vi "Test Asic Rate Scan.vi"(8 "Error IN":errorcluster, 11 "Config Test IN":T2 {"CONFIG GEN"."Vasic Theorical" min=1.0 max=1000000.0 step=1.0 format="%#_6pV"; "CONFIG GEN"."Frequency" min=0.001 max=333000000.0 step=1000.0 format="%#_6pHz"; "CONFIG GEN"."Leading Edge Time" min=1e-09 max=1.0 step=1e-10 format="%#_6ps"; "CONFIG GEN"."Trailing Edge Time" min=1e-09 max=1.0 step=1e-10 format="%#_6ps"; "CONFIG GEN"."Delay" min=0.0 max=1.0 step=1e-12 format="%#_6ps"; "CONFIG GEN"."Trigger Level Sync" items=["ECL", "TTL"]; "CONFIG GEN"."Trigger Sync Out" items=["AB"=3, "B"=2, "A"=1, "None"=0]; "CONFIG GEN"."Load" min=1.0 max=1000000.0 step=1.0 format="%#_6p"; "CONFIG GEN"."DC Offset" min=-10.0 max=10.0 step=0.1 format="%#_6pV"; "CONFIG GEN"."Amplitude" min=0.05 max=5.0 step=0.001 format="%#_6pV"; "CONFIG GEN"."Width Time" min=1.5e-09 max=1.0 step=1e-10 format="%#_6ps"; "CONFIG GEN"."Channel" items=["Channel1"=1, "Channel2"=2]; "Config VGA"."Theoretical Voltage" format="%1.4f"; "Config VGA"."VGA Gain" format="%02x"; "Config VGA"."Frecuency Pulse" format="%0_2p"; "Config VGA"."Pulse Width" format="%04x"; "Config VGA"."Real Voltage" format="%1.5f"; "Config Test"."VALUE IBIAS" max=63 step=1; "Config Test"."Vasic real f.a." min=2.8 max=3.8 step=0.01 format="%.2g"; "Config Test"."Limits Rate Scan adders"."Low" format="%1.3f"; "Config Test"."Limits Rate Scan adders"."High" format="%1.3f"; "Config Test"."Limits ADC"."High" format="%1.4f"; "Config Test"."Limits ADC"."Low" format="%1.3f"; "Config Test"."Lim offset Dig"."Max Dig" format="%.3g"; "Config Test"."Lim Offset Analog"."Min Analog" format="%.3g"; "Config Test"."Lim Offset Analog"."Max Analog" format="%.3g"; "Config Test"."Limits Rate Scan"."Low" format="%1.4f"; "Config Test"."Limits Rate Scan"."High" format="%1.3f"; "Config Test"."Limits Max PN Min NP"."Min P Upper" format="%.3g"; "Config Test"."Limits Max PN Min NP"."Min P Lower" format="%.3g"; "Config Test"."Limits Max PN Min NP"."Max N Lower" format="%.3g"; "Config Test"."Limits Max PN Min NP"."Max N Upper" format="%.3g"; "Config Test"."Limits Max PN Min NP"."Min N Lower" format="%.3g"; "Config Test"."Limits Max PN Min NP"."Min N Upper" format="%.3g"; "Config Test"."Limits Max PN Min NP"."Max P Upper" format="%.3g"; "Config Test"."Limits Max PN Min NP"."Max P Lower" format="%.3g"; "Config Test"."Vasic" min=2.8 max=3.8 step=0.01 format="%.2g"; "Config HW"."Config Rigol DP832"."Channel" items=["+30V Channel 1", "+30V Channel 2", "+5V Channel 3"]; "Config HW"."Config Rigol DP832"."V Limit" format="%.1g"; "Config HW"."Config Rigol DP832"."I Limit" format="%.1g"; "Config HW"."Config Rigol DP832"."V Out" format="%.1g"; "Result"."Test Registros"."Read W/R" format="%04x"; "Result"."Test Registros"."Pattern W/R" format="%04x"; "Result"."Test Registros"."Read Default" format="%04x"; "Result"."Test Registros"."Pattern Default" format="%04x"}) -> (0 "Error OUT":errorcluster={"status"=TRUE, "code"=-1073807343, "source"="VISA Write in Tektronix DPO MSO 2000 4000 Series.lvlib:Auto Scale Math Waveform.vi->TEK_Configura formula Math.vi->Configure osciloscopio FULL con generador.vi->Test Asic Rate Scan.vi->Test Asic V1.0 - copia2019.vi"}, 2 "Rate scan all ok":bool, 3 "Config Test OUT":T2 {"CONFIG GEN"."Vasic Theorical" min=1.0 max=1000000.0 step=1.0 format="%#_6pV"; "CONFIG GEN"."Frequency" min=0.001 max=333000000.0 step=1000.0 format="%#_6pHz"; "CONFIG GEN"."Leading Edge Time" min=1e-09 max=1.0 step=1e-10 format="%#_6ps"; "CONFIG GEN"."Trailing Edge Time" min=1e-09 max=1.0 step=1e-10 format="%#_6ps"; "CONFIG GEN"."Delay" min=0.0 max=1.0 step=1e-12 format="%#_6ps"; "CONFIG GEN"."Trigger Level Sync" items=["ECL", "TTL"]; "CONFIG GEN"."Trigger Sync Out" items=["AB"=3, "B"=2, "A"=1, "None"=0]; "CONFIG GEN"."Load" min=1.0 max=1000000.0 step=1.0 format="%#_6p"; "CONFIG GEN"."DC Offset" min=-10.0 max=10.0 step=0.1 format="%#_6pV"; "CONFIG GEN"."Amplitude" min=0.05 max=5.0 step=0.001 format="%#_6pV"; "CONFIG GEN"."Width Time" min=1.5e-09 max=1.0 step=1e-10 format="%#_6ps"; "CONFIG GEN"."Channel" items=["Channel1"=1, "Channel2"=2]; "Config VGA"."Theoretical Voltage" format="%1.4f"; "Config VGA"."VGA Gain" format="%02x"; "Config VGA"."Frecuency Pulse" format="%0_2p"; "Config VGA"."Pulse Width" format="%04x"; "Config VGA"."Real Voltage" format="%1.5f"; "Config Test"."VALUE IBIAS" max=63 step=1; "Config Test"."Vasic real f.a." min=2.8 max=3.8 step=0.01 format="%.2g"; "Config Test"."Limits Rate Scan adders"."Low" format="%1.3f"; "Config Test"."Limits Rate Scan adders"."High" format="%1.3f"; "Config Test"."Limits ADC"."High" format="%1.4f"; "Config Test"."Limits ADC"."Low" format="%1.3f"; "Config Test"."Lim offset Dig"."Max Dig" format="%.3g"; "Config Test"."Lim Offset Analog"."Min Analog" format="%.3g"; "Config Test"."Lim Offset Analog"."Max Analog" format="%.3g"; "Config Test"."Limits Rate Scan"."Low" format="%1.4f"; "Config Test"."Limits Rate Scan"."High" format="%1.3f"; "Config Test"."Limits Max PN Min NP"."Min P Upper" format="%.3g"; "Config Test"."Limits Max PN Min NP"."Min P Lower" format="%.3g"; "Config Test"."Limits Max PN Min NP"."Max N Lower" format="%.3g"; "Config Test"."Limits Max PN Min NP"."Max N Upper" format="%.3g"; "Config Test"."Limits Max PN Min NP"."Min N Lower" format="%.3g"; "Config Test"."Limits Max PN Min NP"."Min N Upper" format="%.3g"; "Config Test"."Limits Max PN Min NP"."Max P Upper" format="%.3g"; "Config Test"."Limits Max PN Min NP"."Max P Lower" format="%.3g"; "Config Test"."Vasic" min=2.8 max=3.8 step=0.01 format="%.2g"; "Config HW"."Config Rigol DP832"."Channel" items=["+30V Channel 1", "+30V Channel 2", "+5V Channel 3"]; "Config HW"."Config Rigol DP832"."V Limit" format="%.1g"; "Config HW"."Config Rigol DP832"."I Limit" format="%.1g"; "Config HW"."Config Rigol DP832"."V Out" format="%.1g"; "Result"."Test Registros"."Read W/R" format="%04x"; "Result"."Test Registros"."Pattern W/R" format="%04x"; "Result"."Test Registros"."Read Default" format="%04x"; "Result"."Test Registros"."Pattern Default" format="%04x"})   [LabVIEW 2019]
uses:
  Test.ctl
  TEST.TEST CONFIG HW.ctl
  Rigol DP832/DP832_Control Channels.ctl
  TEST.TEST CONFIG TEST MATRIZ.ctl
  TEST.TEST CONFIG TEST.ctl
  TEST.TEST RESULT.ctl
  test_result fvasic.ctl
  TEST.TEST EXECUTION TEST.ctl
  TEST.TEST CONFIG VGA.ctl
  TEST.TEST TEST INFO.ctl
  TEST.TEST INFO PC.ctl
  GenPulse_configurar.ctl
  Global.Salir Ya.vi
panel:
  in  "VISA Tek MDO3104":refnum<visa-resource-name>="USB0::0x0699::0x0408::C016316::INSTR"
  in  "Debug":enum32{"Page 1", "Page 2"}(tab)
  in  "Operacion":enum32{"Page 1", "Page 2"}(tab)
  out "%":u8=9 format="%02d%%"
  out "B":u8(slide)=9 scale=0.0..100.0
  out "Indicador":string="VTheo 0,0500V (Vreal 0,0000V)\nChannel 7 Adder C\nTotal Errors: 0"
  out "Amplitude":dbl
  out "HLTHx":dbl
  out "LLTHx":dbl
  out "WRITE OK":bool
  out "DAC TH0,TH1,TH2 2":u16[][][](array[numeric])
  out "DAC TH3,TH4,TH5 2":u16[][][](array[numeric])
  out "Volt HLTH (salida A)":dbl[][][](array[numeric])
  out "Volt LLTH (salida B)":dbl[][][](array[numeric])
  out "DAC TH0,TH1,TH2":u16
  out "DAC TH3,TH4,TH5":u16
  out "Reference":T1={"Sumador"=2, "Canal"=6, "Tension"=0, "Tension Real"=0.0}
  out "Comparation HLTH":bool[][][](array[boolean])
  out "Comparation LLTH":bool[][][](array[boolean])
  out "Volt HLTH (salida A) corregida":dbl[][][](array[numeric])=[[[nan, nan, nan], [nan, nan, nan], [nan, nan, nan], [nan, nan, nan], [nan, nan, nan], [nan, nan, nan], [nan, nan, nan]]]
  out "HLTH (salida A) cruce por 0":dbl[][](array[numeric])=[[nan, nan, nan], [nan, nan, nan], [nan, nan, nan], [nan, nan, nan], [nan, nan, nan], [nan, nan, nan], [nan, nan, nan]]
  out "Volt LLTH (salida b) corregida":dbl[][][](array[numeric])=[[[nan, nan, nan], [nan, nan, nan], [nan, nan, nan], [nan, nan, nan], [nan, nan, nan], [nan, nan, nan], [nan, nan, nan]]]
  out "LLTH (salida b) cruce por 0":dbl[][](array[numeric])=[[nan, nan, nan], [nan, nan, nan], [nan, nan, nan], [nan, nan, nan], [nan, nan, nan], [nan, nan, nan], [nan, nan, nan]]
  out "HIGH":dbl[](array[numeric])=[0.0593, 0.1073, 0.2039, 0.2977, 0.3918, 0.4828, 0.5702, 0.6594, 0.7367, 0.8087, 0.867]
  out "loW":dbl[](array[numeric])=[0.0264, 0.0665, 0.1423, 0.2207, 0.2962, 0.3691, 0.4392, 0.5107, 0.5726, 0.6304, 0.6771]
  out "Vin asic Theo":dbl[](array[numeric])=[0.05, 0.1, 0.2, 0.3, 0.4, 0.51, 0.6, 0.7, 0.8, 0.9, 1.0]
  out "Vin real gen":dbl[](array[numeric])=[0.054, 0.106, 0.216, 0.322, 0.43, 0.538, 0.648, 0.752, 0.86, 0.966, 1.076]
  # "Vin Asic"
  # "CANAL"
  # "Canal"
  # "VIN ASIC"
  # "Sumador"
  # "Vin Asic"
  # "CANAL"
  # "Canal"
  # "VIN ASIC"
  # "Sumador"
  # "Test ASIC. Rate Scan"
  # "Modo 2\nModo 3\nModo 4\nModo 2\nModo 3\nModo 4"
  # "Modo 2\nModo 3\nModo 4\nModo 2\nModo 3\nModo 4"
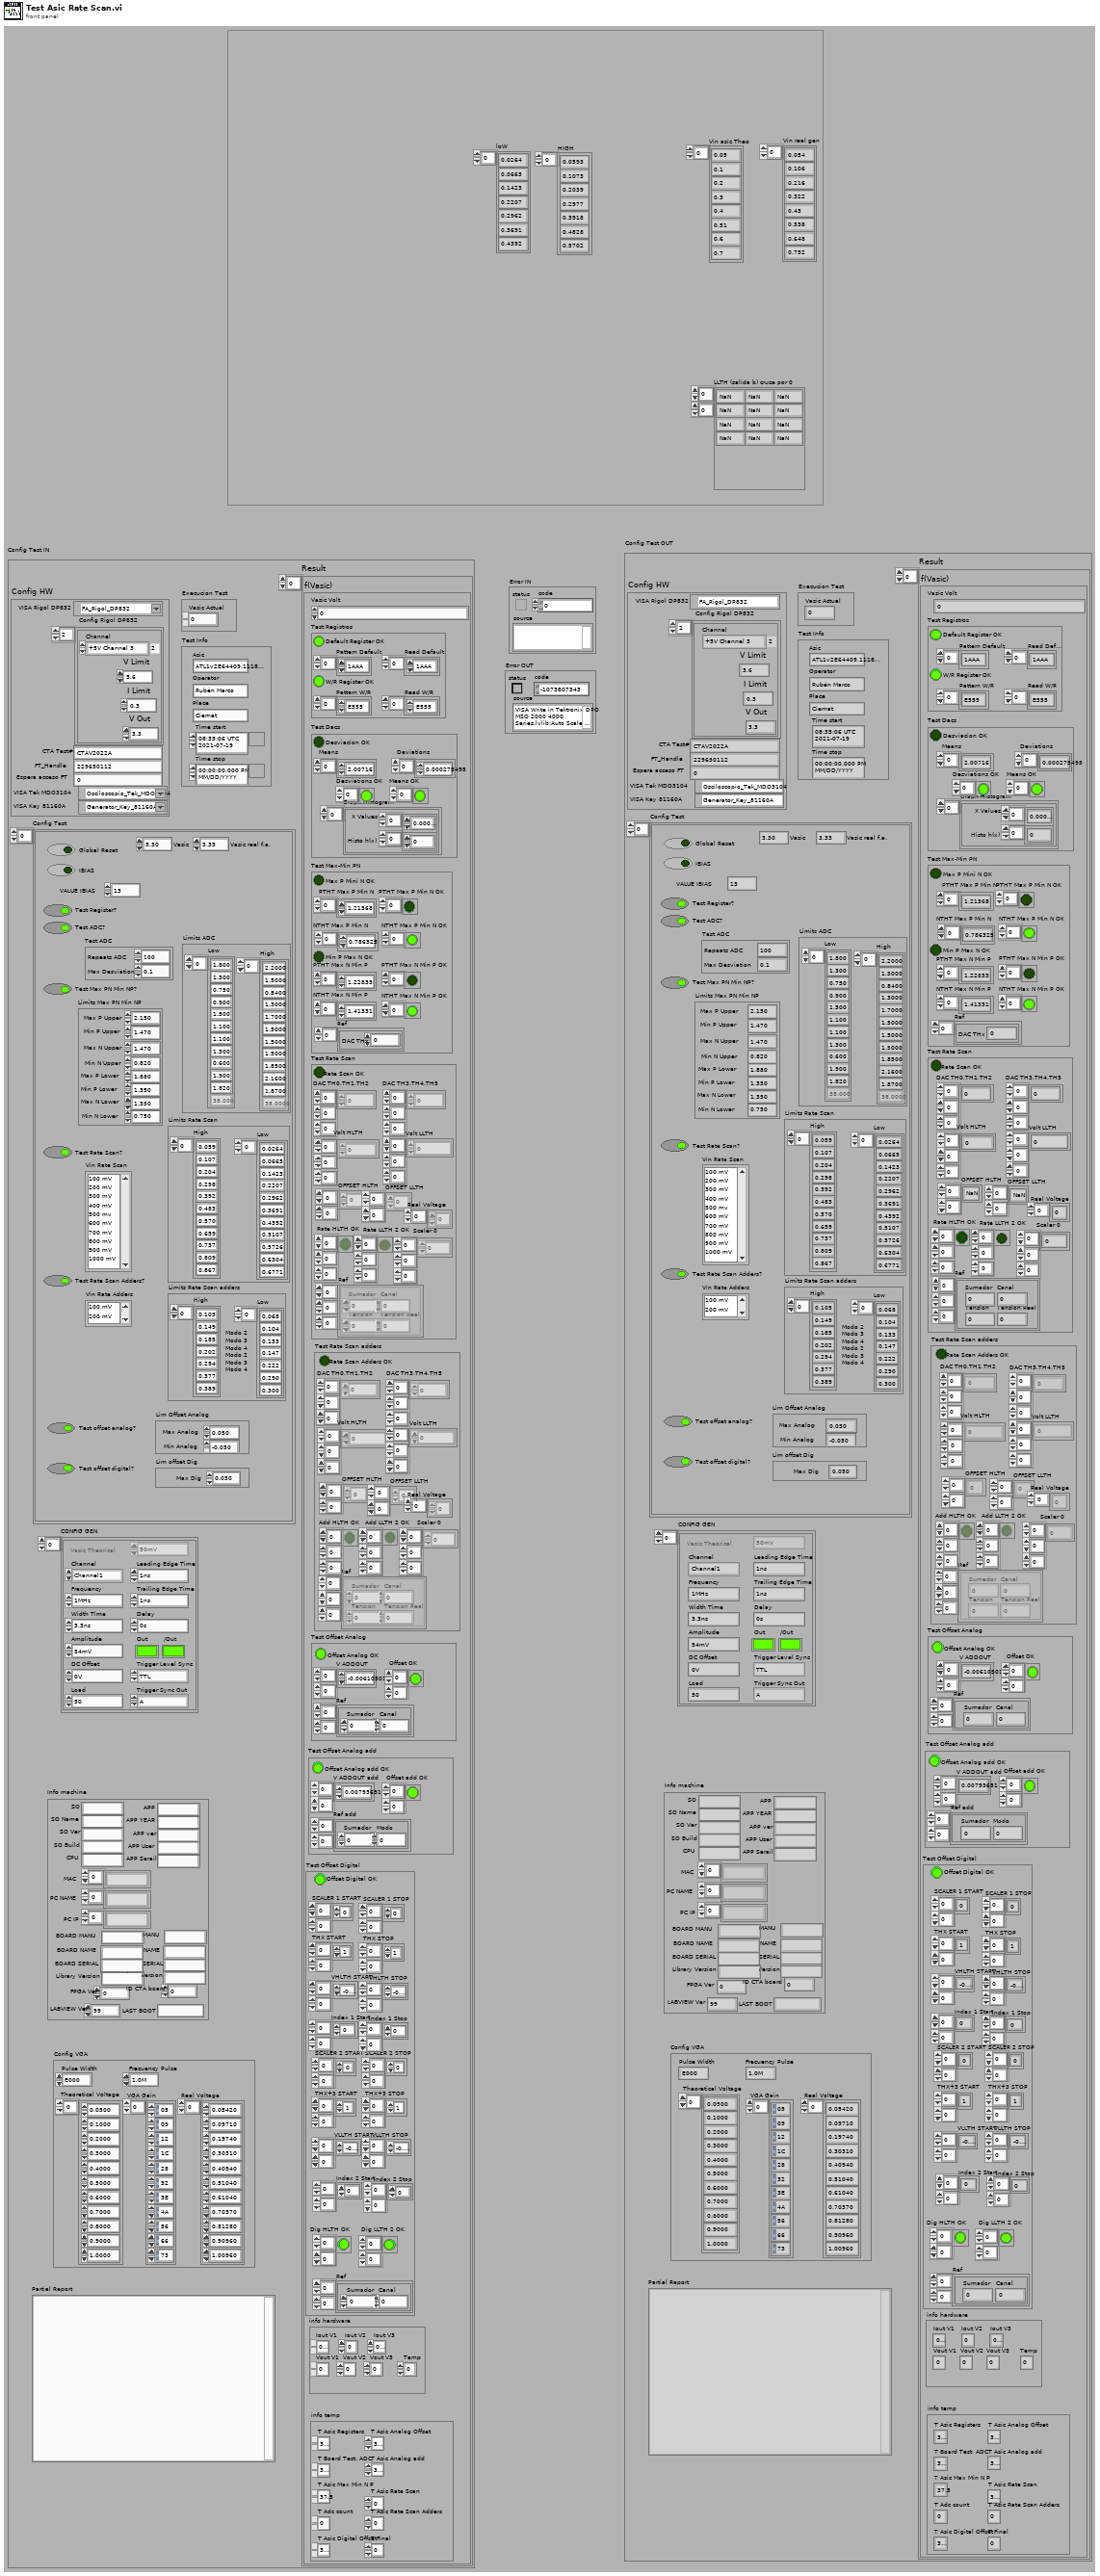
[diagram p1: front panel]
types:
  T1 = cluster{"Sumador":u8, "Canal":u8, "Tension":u8, "Tension Real":dbl}
  T2 = typedef "Test.ctl" = cluster{"Config HW":T3, "Config Test":T5, "Result":T7, "Execucion Test":T9, "Config VGA":T10, "Test Info":T11, "Info machine":T12, "Partial Report":string, "CONFIG GEN":T13[]}
  T3 = typedef "TEST.TEST CONFIG HW.ctl" = cluster{"VISA Rigol DP832":refnum<visa-resource-name>, "Config Rigol DP832":cluster{"Channel":T4, "V Limit":dbl, "I Limit":dbl, "V Out":dbl}[], "CTA Test#":string, "FT_Handle":u32, "Espera acceso FT":u32, "VISA Tek MDO3104":refnum<visa-resource-name>, "VISA Key 81160A":refnum<visa-resource-name>}
  T4 = typedef "DP832_Control Channels.ctl" = i32
  T5 = typedef "TEST.TEST CONFIG TEST MATRIZ.ctl" = T6[]
  T6 = typedef "TEST.TEST CONFIG TEST.ctl" = cluster{"Vasic":dbl, "Global Reset":bool, "Test Register?":bool, "Test ADC?":bool, "Test ADC":cluster{"Repeats ADC":i32, "Max Desviation":dbl}, "Limits ADC":cluster{"Low":dbl[], "High":dbl[]}, "Test Max PN Min NP?":bool, "Limits Max PN Min NP":cluster{"Max P Upper":dbl, "Min P Upper":dbl, "Max N Upper":dbl, "Min N Upper":dbl, "Max P Lower":dbl, "Min P Lower ":dbl, "Max N Lower":dbl, "Min N Lower":dbl}, "Test Rate Scan?":bool, "Vin Rate Scan":i32[], "Limits Rate Scan":cluster{"High":dbl[], "Low":dbl[]}, "Test Rate Scan Adders?":bool, "Vin Rate Adders":i32[], "Limits Rate Scan adders":cluster{"High":dbl[], "Low":dbl[]}, "Test offset analog?":bool, "Lim Offset Analog":cluster{"Max Analog":dbl, "Min Analog":dbl}, "Test offset digital?":bool, "Lim offset Dig":cluster{"Max Dig":dbl}, "Vasic real f.a.":dbl, "IBIAS":bool, "VALUE IBIAS":u8}
  T7 = typedef "TEST.TEST RESULT.ctl" = T8[]
  T8 = typedef "test_result fvasic.ctl" = cluster{"Vasic Volt":i32, "Test Registros":cluster{"Default Register OK":bool, "Pattern Default":u16[], "Read Default":u16[], "W/R Register OK":bool, "Pattern W/R":u16[], "Read W/R":u16[]}, "Test Dacs":cluster{"Desviacion OK":bool, "Means":dbl[], "Deviations":dbl[], "Desviations OK":bool[], "Means OK":bool[], "Graph Histogram":cluster{"X Values":dbl[], "Histo h(x)":i32[]}[]}, "Test Max-Min PN":cluster{"Max P Mini N OK":bool, "PTHT Max P Min N":dbl[], "PTHT Max P Min N OK":bool[], "NTHT Max P Min N":dbl[], "NTHT Max P Min N OK":bool[], "Min P Max N OK":bool, "PTHT Max N Min P":dbl[], "PTHT Max N Min P OK":bool[], "NTHT Max N Min P":dbl[], "NTHT Max N Min P OK":bool[], "Ref":cluster{"DAC THx":u8}[]}, "Test Rate Scan":cluster{"Rate Scan OK":bool, "DAC TH0,TH1,TH2":u16[][][], "Volt HLTH":dbl[][][], "Rate HLTH OK":bool[][][], "DAC TH3,TH4,TH5":u16[][][], "Volt LLTH":dbl[][][], "Rate LLTH 2 OK":bool[][][], "Scaler 0":u16[][][], "Ref":cluster{"Sumador":u8, "Canal":u8, "Tension":u8, "Tension Real":dbl}[][][], "OFFSET HLTH":dbl[][], "OFFSET LLTH":dbl[][], "Real Voltage":dbl[]}, "Test Rate Scan adders":cluster{"Rate Scan Adders OK":bool, "DAC TH0,TH1,TH2":u16[][][], "Volt HLTH":dbl[][][], "Add HLTH OK":bool[][][], "DAC TH3,TH4,TH5":u16[][][], "Volt LLTH":dbl[][][], "Add LLTH 2 OK":bool[][][], "Scaler 0":u16[][][], "Ref":cluster{"Sumador":u8, "Canal":u8, "Tension":u8, "Tension Real":dbl}[][][], "OFFSET HLTH":dbl[][], "OFFSET LLTH":dbl[][], "Real Voltage":dbl[]}, "Test Offset Analog":cluster{"Offset Analog OK":bool, "V ADDOUT":dbl[][], "Offset OK":bool[][], "Ref":cluster{"Sumador":u8, "Canal":u8}[][]}, "Test Offset Digital":cluster{"Offset Digital OK":bool, "SCALER 1 START":u16[][], "SCALER 1 STOP":u16[][], "THX START":u16[][], "THX STOP":u16[][], "VHLTH START":dbl[][], "VHLTH STOP":dbl[][], "Index 1 Start":i32[][], "index 1 Stop":i32[][], "SCALER 2 START":u16[][], "SCALER 2 STOP":u16[][], "THX+3 START":u16[][], "THX+3 STOP":u16[][], "VLLTH START":dbl[][], "VLLTH STOP":dbl[][], "Index 2 Start":i32[][], "index 2 Stop":i32[][], "Dig HLTH OK":bool[][], "Dig LLTH 2 OK":bool[][], "Ref":cluster{"Sumador":u8, "Canal":u8}[][]}, "info hardware":cluster{"Iout V1":dbl, "Iout V2":dbl, "Iout V3":dbl, "Vout V1":dbl, "Vout V2":dbl, "Vout V3":dbl, "Temp":dbl}, "Test Offset Analog add":cluster{"Offset Analog add OK":bool, "V ADDOUT add":dbl[][], "Offset add OK":bool[][], "Ref add":cluster{"Sumador":u8, "Modo":u8}[][]}, "info temp":cluster{"T Asic Registers":dbl, "T Board Test. ADC":dbl, "T Asic Max Min N P":dbl, "T Adc count":dbl, "T Asic Digital Offset":dbl, "T Asic Analog Offset":dbl, "T Asic Analog add":dbl, "T Asic Rate Scan":dbl, "T Asic Rate Scan Adders":dbl, "T Final":dbl}}
  T9 = typedef "TEST.TEST EXECUTION TEST.ctl" = cluster{"Vasic Actual":i32}
  T10 = typedef "TEST.TEST CONFIG VGA.ctl" = cluster{"Theoretical Voltage":dbl[], "Real Voltage":dbl[], "Pulse Width":u16, "Frecuency Pulse":dbl, "VGA Gain":u8[]}
  T11 = typedef "TEST.TEST TEST INFO.ctl" = cluster{"Asic":string, "Operator":string, "Place":string, "Time start":timestamp, "Time stop":timestamp}
  T12 = typedef "TEST.TEST INFO PC.ctl" = cluster{"SO":string, "SO Name":string, "SO Ver":string, "SO Build":string, "CPU":string, "APP":string, "APP YEAR":string, "APP ver":string, "APP User":string, "APP Serail":string, "MAC":string[], "PC NAME":string[], "PC IP":string[], "BIOS MANU":string, "BIOS NAME":string, "BIOS SERIAL":string, "BOARD MANU":string, "BOARD NAME":string, "BOARD SERIAL":string, "Driver Version":string, "Library Version":string, "FPGA Ver":u8, "ID CTA board":u64, "LAST BOOT":string, "LABVIEW Ver":u32}
  T13 = typedef "GenPulse_configurar.ctl" = cluster{"Channel":u16, "Frequency":dbl, "Width Time":dbl, "Amplitude":dbl, "DC Offset":dbl, "Load":dbl, "Leading Edge Time":dbl, "Trailing Edge Time":dbl, "Delay":dbl, "Out":bool, "/Out":bool, "Trigger Level Sync":u16, "Trigger Sync Out":u16, "Vasic Theorical":dbl}
  T14 = enum16{"Always On", "Always Off", "Off While Running"}
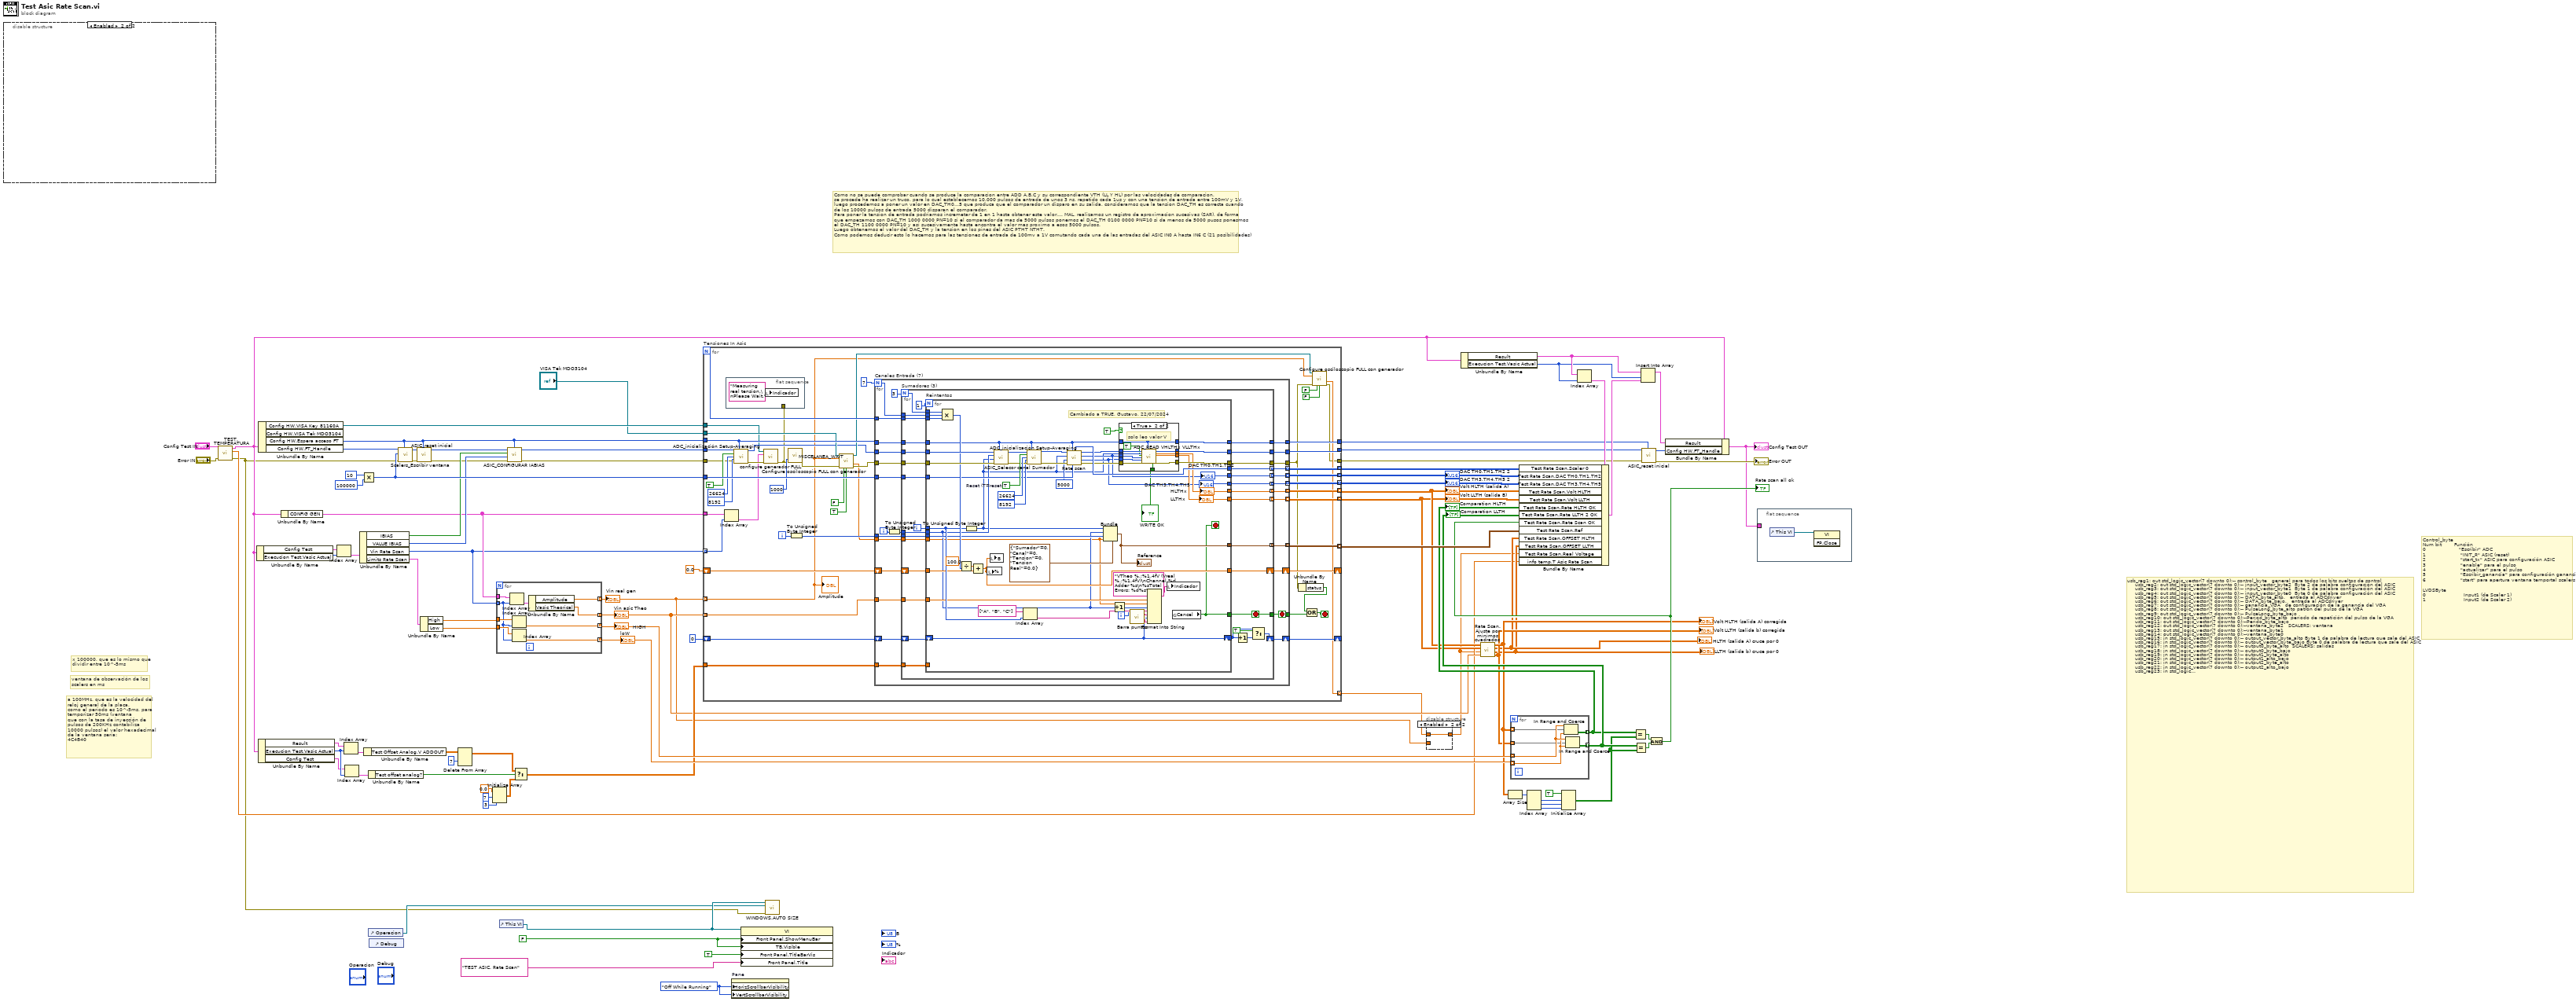
[diagram p0: block diagram]
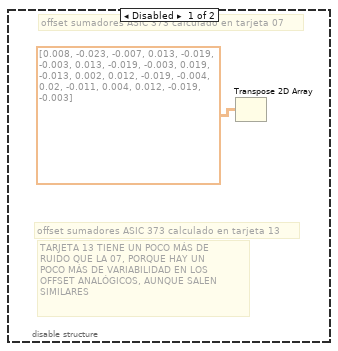
[diagram p3: hidden frame]
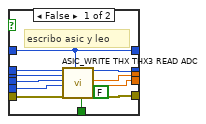
[diagram p4: hidden frame]
diagram:
  w22 = T14."Off While Running" ("Horizontal Scrollbar Visibility")
  w53 = FALSE ("Front Panel Window:Show Menu Bar")
  # "Como no se puede comprobar cuando se produce la comparacion entre ADD A,B,C y su correspondiente VTH (LL Y HL) por las velocidades de comparacion,\nse procede ha realizar un truco, para lo cual establecemos 10.000 pulsos de entrada de unos 3 ns, repetido cada 1us y con una tension de entrada entre 100mV y 1V,\nluego procedemos a poner un valor en DAC_TH0...5 que produca que el comparador un disparo en su salida, consideramos que la tension DAC_TH es correcta cuando\nde los 10000 pulsos de entrada 5000 disparan el comparador.\nPara poner la tension de entrada podriamos incremetar de 1 en 1 hasta obtener este valor.... MAL. realizamos un registro de aproximacion sucesivas (SAR), de forma\nque empezamos con DAC_TH 1000 0000 PN=10 si el comparador da mas de 5000 pulsos ponemos el DAC_TH 0100 0000 PN=10 si da menos de 5000 pusos ponesmos\nel DAC_TH 1100 0000 PN=10 y asi sucesivamente hasta encontra el valor mas proximo a esos 5000 pulsos. \nLuego obtenemos el valor del DAC_TH y la tension en los pines del ASIC PTHT NTHT.\nComo podemos deducir esto lo hacemos para las tensiones de entrada de 100mv a 1V comutando cada una de las entradas del ASIC IN0 A hasta IN6 C (21 posibilidades)"
  # "Control_byte\nNum bit        Función\n0                     \"Escribir\" ADC\n1                      \"INIT_R\" ASIC (reset)\n2                      \"start_tx\" ASIC para configuración ASIC\n3                      \"enable\" para el pulso\n4                      \"actualizar\" para el pulso\n5                      \"Escribir_ganancia\" para configuración ganancia\n6                      \"start\" para apertura ventana temportal scalers\n\nLVDSByte\n0                        Input1 (de Scaler 1)\n1                        Input2 (de Scaler 2)"
  # "usb_reg1: out std_logic_vector(7 downto 0);-- control_byte\t\t\tgeneral para todos los bits sueltos de control\n\t\t\t  usb_reg2: out std_logic_vector(7 downto 0);-- input_vector_byte2 \tByte 2 de palabra configuración del ASIC\n\t\t\t  usb_reg3: out std_logic_vector(7 downto 0);-- input_vector_byte1 \tByte 1 de palabra configuración del ASIC\n\t\t\t  usb_reg4: out std_logic_vector(7 downto 0);-- input_vector_byte0 \tByte 0 de palabra configuración del ASIC\n\t\t\t  usb_reg5: out std_logic_vector(7 downto 0);-- DATA_byte_alto, \t\tentrada al ADCdriver\n\t\t\t  usb_reg6: out std_logic_vector(7 downto 0);-- DATA_byte_bajo, \t\tentrada al ADCdriver\n\t\t\t  usb_reg7: out std_logic_vector(7 downto 0);-- ganancia_VGA\t\t\tde configuración de la ganancia del VGA\n\t\t\t  usb_reg8: out std_logic_vector(7 downto 0);-- PulseLong_byte_alto\tpatrón del pulso de la VGA\n\t\t\t  usb_reg9: out std_logic_vector(7 downto 0);-- PulseLong_byte_bajo\n\t\t\t  usb_reg10: out std_logic_vector(7 downto 0);--Period_byte_alto\t\tperíodo de repetición del pulso de la VGA\n\t\t\t  usb_reg11: out std_logic_vector(7 downto 0);--Perido_byte_bajo\n\t\t\t  usb_reg12: out std_logic_vector(7 downto 0);--ventana_byte2\t\t\tSCALERS: ventana\n\t\t\t  usb_reg13: out std_logic_vector(7 downto 0);--ventana_byte1\t\n\t\t\t  usb_reg14: out std_logic_vector(7 downto 0);--ventana_byte0\n\t\t\t  usb_reg15: in std_logic_vector(7 downto 0);-- output_vector_byte_alto\tByte 1 de palabra de lectura que sale del ASIC\n\t\t\t  usb_reg16: in std_logic_vector(7 downto 0);-- output_vector_byte_bajo\tByte 0 de palabra de lectura que sale del ASIC\n\t\t\t  usb_reg17: in std_logic_vector(7 downto 0);-- output0_byte_alto\t\tSCALERS: salidas\n\t\t\t  usb_reg18: in std_logic_vector(7 downto 0);-- output0_byte_bajo\n\t\t\t  usb_reg19: in std_logic_vector(7 downto 0);-- output1_byte_alto\n\t\t\t  usb_reg20: in std_logic_vector(7 downto 0);-- output1_alto_bajo \n\t\t\t  usb_reg21: in std_logic_vector(7 downto 0);-- output2_byte_alto \n\t\t\t  usb_reg22: in std_logic_vector(7 downto 0);-- output2_alto_bajo \n\t\t\t  usb_reg23: in std_logic_vector(7 downto 0);-- para el canal_0 del ADCdriver\n\t\t\t  usb_reg24: in std_logic_vector(7 downto 0);\n\t\t\t  usb_reg25: in std_logic_vector(7 downto 0);-- para el canal_1 del ADCdriver\n\t\t\t  usb_reg26: in std_logic_vector(7 downto 0);\n\t\t\t  usb_reg27: in std_logic_vector(7 downto 0);-- para el canal_2 del ADCdriver\n\t\t\t  usb_reg28: in std_logic_vector(7 downto 0);\n\t\t\t  usb_reg29: in std_logic_vector(7 downto 0);-- para el canal_3 del ADCdriver\n\t\t\t  usb_reg30: in std_logic_vector(7 downto 0);\n\t\t\t  usb_reg31: in std_logic_vector(7 downto 0);-- para el canal_4 del ADCdriver\n\t\t\t  usb_reg32: in std_logic_vector(7 downto 0);\n\t\t\t  usb_reg33: in std_logic_vector(7 downto 0);-- para el canal_5 del ADCdriver\n\t\t\t  usb_reg34: in std_logic_vector(7 downto 0);\n\t\t\t  usb_reg35: in std_logic_vector(7 downto 0);-- para el canal_6 del ADCdriver\n\t\t\t  usb_reg36: in std_logic_vector(7 downto 0);\n\t\t\t  usb_reg37: in std_logic_vector(7 downto 0);-- para el canal_7 del ADCdriver\n\t\t\t  usb_reg38: in std_logic_vector(7 downto 0);\n\t\t\t  usb_reg39: in std_logic_vector(7 downto 0);-- para el canal_8 del ADCdriver\n\t\t\t  usb_reg40: in std_logic_vector(7 downto 0);\n\t\t\t  usb_reg41: in std_logic_vector(7 downto 0);-- para el canal_9 del ADCdriver\n\t\t\t  usb_reg42: in std_logic_vector(7 downto 0);\n\t\t\t  usb_reg43: in std_logic_vector(7 downto 0);-- para el canal_10 del ADCdriver\n\t\t\t  usb_reg44: in std_logic_vector(7 downto 0)--;  \n\n     usb_reg55 => LVDSByte"
  # "x 100000, que es lo mismo que dividir entre 10^-5ms"
  # "ventana de observación de los scalers en ms"
  # "a 100MHz, que es la velocidad del reloj general de la placa,\ncomo el período es 10^-5ms, para temporizar 50ms (ventana \nque con la tasa de inyección de pulsos de 200KHz contabiliza \n10000 pulsos) el valor hexadecimal de la ventana sería:\n4C4B40"
  n1 = disable-structure shown="Enabled" {
    frame Disabled {
      # "TARJETA 13 TIENE UN POCO MÁS DE \nRUIDO QUE LA 07, PORQUE HAY UN\nPOCO MÁS DE VARIABILIDAD EN LOS \nOFFSET ANALÓGICOS, AUNQUE SALEN\nSIMILARES"
      # "offset sumadores ASIC 373 calculado en tarjeta 13"
      # "offset sumadores ASIC 373 calculado en tarjeta 07"
      n2 = Transpose 2D Array(2D array=dbl[][] [[0.008, -0.023, -0.007], [0.013, -0.019, -0.003], [0.013, -0.019, -0.003], [0.019, -0.013, 0.002], [0.012, -0.019, -0.004], [0.02, -0.011, 0.004], [0.012, -0.019, -0.003]]) -> ()  [unwired: 1 out]
    }
    frame Enabled {
    }
  }
  n3 = call "TEST.TEMPERATURA.vi"("error IN"="Error IN", "input cluster"="Config Test IN") -> ("error out"=w4:errorcluster, "Temperatura"=w10:dbl, "OUT cluster 2"=w11:T2)  [unwired: 7 in]
  n4 = Unbundle By Name(w11) -> ("Config Test"=w76:T5, "Execucion Test.Vasic Actual"=w75:i32)
  n5 = Unbundle By Name(w11) -> ("Result"=w39:T7, "Execucion Test.Vasic Actual"=w35:i32, "Config Test"=w32:T5)
  n6 = Unbundle By Name(w11) -> ("Config HW.VISA Key 81160A"=w6:refnum<visa-resource-name>, "Config HW.Espera acceso FT"=w42:u32, "Config HW.FT_Handle"=w5:u32)  [unwired: 1 out]
  n7 = Unbundle By Name(w11) -> ("CONFIG GEN"=w3:T13[])
  n8 = Index Array(array=w76, index=w75) -> (element=w74:T6)
  n9 = Index Array(array=w39, index=w35) -> (element=w38:T8)
  n10 = Index Array(array=w32, index=w35) -> (element=w34:T6)
  n11 = Unbundle By Name(w74) -> ("IBIAS"=w44:bool, "VALUE IBIAS"=w43:u8, "Vin Rate Scan"=w2:i32[], "Limits Rate Scan"=w62:cluster{"High":dbl[], "Low":dbl[]})
  n12 = Multiply(x=u32 10 ("Ventana"), y=u32 100000 ("Ventana")) -> (x*y=w84:u32)
  n13 = Unbundle By Name(w38) -> ("Test Offset Analog.V ADDOUT"=w36:dbl[][])
  n14 = control-ref of="Operacion"() -> (w14:refnum<vi>)
  n15 = Unbundle By Name(w34) -> ("Test offset analog?"=w31:bool)
  n16 = control-ref of="Debug"() -> ()  [unwired: 1 out]
  n17 = call "Scalers_Escribir ventana.vi"("Espera acceso USB"=w42, "error in"=w4, "Ventana"=w84, "ftHandle_in"=w5) -> ("error out"=w85:errorcluster, "ftHandle_out"=w86:u32)  [unwired: 6 in]
  n18 = call "ASIC_reset inicial.vi"("Espera acceso USB"=w42, "error in"=w85, "ftHandle_in"=w86) -> ("error out"=w41:errorcluster, "ftHandle_out"=w83:u32)  [unwired: 7 in]
  n19 = Unbundle By Name(w62) -> ("High"=w61:dbl[], "Low"=w60:dbl[])
  n20 = Delete From Array(array=w36, index (row)=7) -> (array with subset deleted=w26:dbl[][])  [unwired: 2 in, 1 out]
  n21 = Initialize Array(0.0, 7 ("dimension size"), 3 ("dimension size")) -> (w27:dbl[][])
  n22 = for {
    tunnel: w2 -> [w94] mode=indexing
    tunnel: [w92] -> w9 mode=indexing
    tunnel: w61 -> [w98]
    tunnel: w60 -> [w97]
    tunnel: [w96] -> w48 mode=indexing
    tunnel: [w95] -> w47 mode=indexing
    tunnel: [w91] -> w21 mode=indexing
    tunnel: w3 -> [w90]
    n23 = Index Array(array=w90, index=w94) -> (element=w93:T13)
    n24 = Index Array(array=w97, index=w94) -> (element=w95:dbl)
    n25 = Index Array(array=w98, index=w94) -> (element=w96:dbl)
    n26 = Unbundle By Name(w93) -> ("Amplitude"=w92:dbl, "Vasic Theorical"=w91:dbl)
  }
  "HIGH" <- w48
  "loW" <- w47
  "Vin asic Theo" <- w21
  "Vin real gen" <- w9
  n27 = control-ref of="This VI"() -> (w50:refnum<vi>)
  n28 = call "ASIC_CONFIGURAR IABIAS.vi"("Espera acceso USB"=w42, "error in"=w41, "IBIAS VALUE"=w43, "IBIAS"=w44, "ftHandle_in"=w83) -> ("error out"=w40:errorcluster, "ftHandle_out"=w45:u32)  [unwired: 5 in]
  n29 = Select(t=w26, s=w31, f=w27) -> (s? t:f=w25:dbl[][])
  n30 = for "Tensiones In Asic" {
    N -> [w129]
    tunnel: w42 -> [w138]
    tunnel: w84 -> [w147]
    tunnel: [w144] -> w23 mode=indexing
    tunnel: [w143] -> w81 mode=indexing
    tunnel: [w136] -> w20 mode=indexing
    tunnel: [w135] -> w19 mode=indexing
    tunnel: w9 -> [w103] mode=indexing
    tunnel: [w133] -> w73 mode=indexing
    tunnel: [w131] -> w65 mode=indexing
    tunnel: [w130] -> w54
    tunnel: w21 -> [w102] mode=indexing
    shift-right: [w127] -> _
    shift-left: 0.0 ("x/y") -> [w128]
    shift-right: [w125] -> _
    shift-left: u32 0 ("ms wait IN") -> [w126]
    tunnel: w25 -> [w124]
    tunnel: w45 -> [w139]
    tunnel: [w145] -> w55
    tunnel: w40 -> [w137]
    tunnel: [w117] -> w58
    tunnel: "VISA Tek MDO3104" -> [w113]
    tunnel: [w118] -> w8 mode=indexing
    tunnel: w6 -> [w104]
    tunnel: w3 -> [w101]
    tunnel: w2 -> [w99] mode=indexing
    i -> [w134]
    stop <- w108 stop-if-true
    n31 = Index Array(array=w101, index=w99) -> (element=w100:T13)
    n32 = flat-sequence {
      tunnel: w105 -> [_]
      frame #0 {
        n33 = local write "Indicador"("Measuring real tension.\nPlease Wait." ("Indicador")) -> ()
      }
    }
    n34 = call "ADC_inicialización Setup-Averaging.vi"("ftHandle_in 2"=w139, "Espera acceso USB"=w138, "Reset (T=reset)"=TRUE, "Registro Setup (0x6800)"=u16 26624, "Registro Averaging (0x3200)"=u16 8192 ("Registro Setup (0x6800)"), "error in 2"=w137) -> ("ftHandle_out"=w107:u32, "error out"=w106:errorcluster)  [unwired: 8 in]
    n35 = call "configure generador FULL.vi"("error in"=w106, "Config Pulse"=w100, "VISA Key 81160A"=w104) -> ("error out"=w105:errorcluster)  [unwired: 6 in, 2 out]
    n36 = call "MISCELANEA_WAIT.vi"("ms wait IN"=u32 1000, "Error IN"=w105) -> ("Error OUT"=w122:errorcluster)  [unwired: 16 in, 1 out]
    n37 = To Unsigned Byte Integer(number=w134) -> (unsigned 8bit integer=w132:u8)
    n38 = call "Configure osciloscopio FULL con generador.vi"("Visa MDO3104"=w113, "Amplitud"=w103, "error out"=w122, "Esperar a completar estadisticas"=FALSE ("Wait medida"), "Configurar Osciloscopio"=TRUE ("Solo Medida")) -> ("VISA resource name out 2"=w112:refnum<visa-resource-name>, "Math (CH1-CH2)"=w119:dbl, "error out 2"=w121:errorcluster)  [unwired: 6 in, 2 out]
    n39 = for "Canales Entrada (7)" {
      N: 7 -> [w157]
      tunnel: w138 -> [w171]
      tunnel: w147 -> [w172]
      tunnel: [w166] -> w144 mode=indexing
      tunnel: [w165] -> w143 mode=indexing
      tunnel: [w164] -> w136 mode=indexing
      tunnel: [w163] -> w135 mode=indexing
      tunnel: w132 -> [w162]
      tunnel: w119 -> [w161]
      tunnel: [w160] -> w133 mode=indexing
      tunnel: [w159] -> w131 mode=indexing
      tunnel: [w158] -> w130
      tunnel: w129 -> [w156]
      tunnel: w102 -> [w155]
      shift-right: [w153] -> w127
      shift-left: w128 -> [w154]
      tunnel: [w152] -> w109
      shift-right: [w150] -> w125
      shift-left: w126 -> [w151]
      tunnel: w124 -> [w149]
      tunnel: w107 -> [w175]
      tunnel: [w168] -> w145
      tunnel: w121 -> [w174]
      tunnel: [w167] -> w111
      i -> [w173]
      stop <- w152 stop-if-true
      n40 = To Unsigned Byte Integer(number=w173) -> (unsigned 8bit integer=w169:u8)
      n41 = for "Sumadores (3)" {
        N: 3 -> [w196]
        tunnel: w169 -> [w192]
        tunnel: w172 -> [w204]
        tunnel: w171 -> [w198]
        tunnel: [w206] -> w166 mode=indexing
        tunnel: [w205] -> w165 mode=indexing
        tunnel: [w187] -> w164 mode=indexing
        tunnel: [w186] -> w163 mode=indexing
        tunnel: w162 -> [w197]
        tunnel: w161 -> [w193]
        tunnel: [w200] -> w160 mode=indexing
        tunnel: [w199] -> w159 mode=indexing
        tunnel: [w179] -> w158
        tunnel: w157 -> [w195]
        tunnel: w156 -> [w194]
        tunnel: w155 -> [w190]
        shift-right: [w188] -> w153
        shift-left: w154 -> [w189]
        tunnel: [w183] -> w152
        shift-right: [w182] -> w150
        shift-left: w151 -> [w184]
        tunnel: w149 -> [w178]
        tunnel: w175 -> [w202]
        tunnel: [w201] -> w168
        tunnel: w174 -> [w203]
        tunnel: [w176] -> w167
        i -> [w191]
        stop <- w183 stop-if-true
        n42 = for "Reintentos" {
          N: 1 -> [_]
          tunnel: [w215] -> w206
          tunnel: [w214] -> w205
          tunnel: w204 -> [w223]
          tunnel: w202 -> [w252]
          tunnel: [w249] -> w201
          tunnel: [w246] -> w200
          tunnel: [w245] -> w199
          tunnel: w198 -> [w222]
          tunnel: w197 -> [w221]
          tunnel: w196 -> [w243]
          tunnel: w195 -> [w242]
          tunnel: w194 -> [w241]
          tunnel: w193 -> [w208]
          tunnel: w192 -> [w211]
          tunnel: w191 -> [w237]
          tunnel: w190 -> [w234]
          tunnel: [w209] -> w183
          tunnel: [w228] -> w187
          tunnel: [w227] -> w186
          tunnel: w189 -> [w231]
          tunnel: [w229] -> w188
          shift-right: [w224] -> w181
          shift-left: w184 -> [w224]
          tunnel: [w213] -> w179
          tunnel: w178 -> [_]
          tunnel: w203 -> [w253]
          tunnel: [w248] -> w176
          i -> [w226]
          stop <- w209 stop-if-true
          w255 = TRUE  # Reset (T=reset)
          # "Cambiado a TRUE, Gustavo, 22/07/2024"
          n43 = Compound Arithmetic op=MULTIPLY(w243, w242, w241) -> (w240:i32)
          n44 = Divide(x=100.0, y=w240) -> (x/y=w230:dbl)
          n45 = To Unsigned Byte Integer(number=w237) -> (unsigned 8bit integer=w210:u8)
          n46 = Add(x=w230, y=w231) -> (x+y=w229:dbl)
          n47 = local write "%"(w229) -> ()
          n48 = local write "B"(w229) -> ()
          n49 = call "ASIC_Selecor canal Sumador.vi"("Espera acceso USB"=w222, "error in"=w253, "Sumador"=w210, "Canal"=w211, "ftHandle_in"=w252) -> ("error out"=w251:errorcluster, "ftHandle_out"=w250:u32)  [unwired: 4 in, 1 out]
          n50 = Index Array(array=string[] ["A", "B", "C"], index=w237) -> (element=w236:string)
          n51 = call "ADC_inicialización Setup-Averaging.vi"("ftHandle_in 2"=w250, "Espera acceso USB"=w222, "Reset (T=reset)"=w255, "Registro Setup (0x6800)"=u16 26624, "Registro Averaging (0x3200)"=u16 8192 ("Registro Setup (0x6800)"), "error in 2"=w251) -> ("ftHandle_out"=w220:u32, "error out"=w219:errorcluster)  [unwired: 8 in]
          n52 = call "Rate scan.vi"("T Ventana"=w223, "Espera acceso USB"=w222, "error in 2"=w219, "Valor buscado scalers (5000)"=u16 5000 ("Valor buscado scalers"), "Sumador"=w210, "ftHandle_in 2"=w220) -> ("error out 2"=w217:errorcluster, "DAC\nTH3,TH4,TH5"=w214:u16, "DAC\nTH0,TH1,TH2"=w215:u16, "ftHandle_out 2"=w218:u32, "Scaler 1"=w246:u16)  [unwired: 1 in]
          "DAC TH0,TH1,TH2" <- w215
          "DAC TH3,TH4,TH5" <- w214
          n53 = Bundle(cluster=T1 {"Sumador"=0, "Canal"=0, "Tension"=0, "Tension Real"=0.0}, "Sumador"=w210, "Canal"=w211, "Tension"=w221, "Tension Real"=w208) -> (w245:T1)
          "Reference" <- w245
          n54 = Increment(x=w211) -> (x+1=w233:u8)
          n55 = case shown="True" TRUE {
            tunnel: [w266 w278] -> w249
            tunnel: [w260 w277] -> w248
            tunnel: [w258 w276] -> w228
            tunnel: [w259 w275] -> w227
            tunnel: w222 -> [w257 w268]
            tunnel: w210 -> [w264 w274]
            tunnel: w218 -> [w265 w273]
            tunnel: w217 -> [w261 w272]
            tunnel: w215 -> [w263 w271]
            tunnel: w214 -> [w262 w270]
            tunnel: [w257 w268] -> w213
            tunnel: [FALSE ("WRITE OK") w267] -> w207
            frame False {
              # "escribo asic y leo"
              n56 = call "ASIC_WRITE THX THX3 READ ADC.vi"("ftHandle_in"=w265, "Sumador"=w264, "THX"=w263, "THX+3"=w262, "error in"=w261, "Espera acceso USB 2"=w257) -> ("ftHandle_out"=w266:u32, "HLTHx"=w258:dbl, "LLTHx"=w259:dbl, "error out"=w260:errorcluster)  [unwired: 10 in]
            }
            frame True {
              # "solo leo valor V"
              n57 = call "ADC_READ VHLTHx VLLTHx.vi"("ftHandle_out 2"=w273, "Sumador"=w274, "referenciar"=TRUE, "ref DAC\nTH0,TH1,TH2"=w271, "ref DAC\nTH3,TH4,TH5"=w270, "error out 2"=w272, "Espera acceso FT"=w268) -> ("WRITE OK"=w267:bool, "ftHandle_out"=w278:u32, "HLTHx"=w276:dbl, "LLTHx"=w275:dbl, "error out"=w277:errorcluster)  [unwired: 8 in]
            }
          }
          "HLTHx" <- w228
          "LLTHx" <- w227
          "WRITE OK" <- w207
          n58 = call "Barra puntos.vi"("#N"=w226) -> ("String"=w225:string)  [unwired: 8 in]
          n59 = Format Into String(format string="VTheo %,;%1.4fV (Vreal %,;%1.4fV)\nChannel %d Adder %s\n%sTotal Errors: %d%s", w234, w208, w233, w236, w225, w224, w225) -> (resulting string=w235:string)  [unwired: 2 in, 1 out]
          n60 = local write "Indicador"(w235) -> ()
          n61 = global read "Global.Salir Ya.vi" "Cancel"() -> (w209:bool)
        }
        n62 = Increment(x=w181) -> (x+1=w180:u32)
        n63 = Select(t=w181, s=TRUE, f=w180) -> (s? t:f=w182:u32)
      }
    }
    n64 = Unbundle By Name(w111) -> ("status"=w110:bool)
    n65 = Compound Arithmetic op=OR(w110, w109) -> (w108:bool)
    n66 = call "Configure osciloscopio FULL con generador.vi"("Visa MDO3104"=w112, "Amplitud"=w103, "error out"=w111, "Esperar a completar estadisticas"=FALSE, "Configurar Osciloscopio"=FALSE ("Solo Medida")) -> ("Math (CH1-CH2)"=w118:dbl, "error out 2"=w117:errorcluster)  [unwired: 6 in, 3 out]
    "Amplitude" <- w103
  }
  "DAC TH0,TH1,TH2 2" <- w23
  "DAC TH3,TH4,TH5 2" <- w81
  "Volt HLTH (salida A)" <- w20
  "Volt LLTH (salida B)" <- w19
  n67 = property on="Pane" class="Pane"("HorizScrollbarVisibility"=w22, "VertScrollbarVisibility"=w22) -> ()  [unwired: 2 in, 2 out]
  n68 = property class="VI"(reference=w50, "Front Panel.ShowMenuBar"=w53, "TB.Visible"=w53, "Front Panel.TitleBarVis"=TRUE ("Front Panel Window:Title Bar Visible"), "Front Panel.Title"="TEST ASIC. Rate Scan" ("Front Panel Window:Title")) -> ()  [unwired: 1 in, 2 out]
  n69 = call "WINDOWS.AUTO SIZE.vi"("Error In"=w4, "TAB.AutoAjuste"=w14, "This VI"=w50) -> ()  [unwired: 4 in, 1 out]
  n70 = disable-structure shown="Enabled" {
    disable-tunnel: w9 -> [w279 _]
    disable-tunnel: [w279 w280] -> w7
    disable-tunnel: w8 -> [_ w280]
    frame Disabled {
    }
    frame Enabled {
    }
  }
  n71 = Unbundle By Name(w11) -> ("Result"=w79:T7, "Execucion Test.Vasic Actual"=w78:i32)
  n72 = call "Rate Scan. Ajuste por minimos cuadrados.vi"("V asic Theorical"=w21, "V asic Real"=w7, "Salida B"=w19, "Salida A"=w20) -> ("Salida B rectificada"=w17:dbl[][][], "Cruze por 0 Salida B"=w15:dbl[][], "Cruze por 0 Salida A"=w16:dbl[][], "Salida A rectificada"=w18:dbl[][][])
  "Volt HLTH (salida A) corregida" <- w18
  "HLTH (salida A) cruce por 0" <- w16
  "Volt LLTH (salida b) corregida" <- w17
  "LLTH (salida b) cruce por 0" <- w15
  n73 = Array Size(array=w18) -> (size(s)=w72:i32[])
  n74 = for {
    tunnel: w18 -> [w282] mode=indexing
    tunnel: w17 -> [w281] mode=indexing
    tunnel: [w285] -> w24 mode=indexing
    tunnel: [w286] -> w63 mode=indexing
    tunnel: w48 -> [w284] mode=indexing
    tunnel: w47 -> [w283] mode=indexing
    n75 = In Range and Coerce(upper limit=w284, x=w282, lower limit=w283) -> (In Range?=w285:bool[][])  [unwired: 1 out]
    n76 = In Range and Coerce(upper limit=w284, x=w281, lower limit=w283) -> (In Range?=w286:bool[][])  [unwired: 1 out]
  }
  "Comparation HLTH" <- w24
  "Comparation LLTH" <- w63
  n77 = Index Array(array=w72) -> (element #1=w71:i32, element #2=w70:i32, element #3=w69:i32)  [unwired: 3 in]
  n78 = Initialize Array(TRUE, w71, w70, w69) -> (w59:bool[][][])
  n79 = Index Array(array=w79, index=w78) -> (element=w82:T8)
  n80 = Equal?(x=w24, y=w59) -> (x = y?=w67:bool)
  n81 = Equal?(x=w63, y=w59) -> (x = y?=w66:bool)
  n82 = call "ASIC_reset inicial.vi"("Espera acceso USB"=w54, "error in"=w58, "ftHandle_in"=w55) -> ("error out"=→"Error OUT":errorcluster, "ftHandle_out"=w56:u32)  [unwired: 7 in]
  n83 = And(x=w67, y=w66) -> (x .and. y?=w64:bool)
  "Rate scan all ok" <- w64
  n84 = Bundle By Name(cluster=w82, "Test Rate Scan.Scaler 0"=w73, "Test Rate Scan.DAC TH0,TH1,TH2"=w23, "Test Rate Scan.DAC TH3,TH4,TH5"=w81, "Test Rate Scan.Volt HLTH"=w20, "Test Rate Scan.Volt LLTH"=w19, "Test Rate Scan.Rate HLTH OK"=w24, "Test Rate Scan.Rate LLTH 2 OK"=w63, "Test Rate Scan.Rate Scan OK"=w64, "Test Rate Scan.Ref"=w65, "Test Rate Scan.OFFSET HLTH"=w16, "Test Rate Scan.OFFSET LLTH"=w15, "Test Rate Scan.Real Voltage"=w7, "info temp.T Asic Rate Scan"=w10) -> (w80:T8)
  n85 = Insert Into Array(array=w79, index=w78, new element=w80) -> (w77:T7)
  n86 = Bundle By Name(cluster=w11, "Result"=w77, "Config HW.FT_Handle"=w56) -> (w33:T2)
  "Config Test OUT" <- w33
  n87 = flat-sequence {
    tunnel: w33 -> [_]
    frame #0 {
      n88 = control-ref of="This VI"() -> (w287:refnum<vi>)
      n89 = invoke class="VI" method="FP.Close"(reference=w287) -> ()  [unwired: 2 in, 3 out]
    }
  }
